vi "build_pck.vi"(8 "data in":u8[](array[numeric])=[0, 0, 0, 0], 9 "dev_id":u32, 10 "pck_num":u32, 11 "cmd_type":T1) -> (3 "w5500_pck":T2)   [LabVIEW 2021]
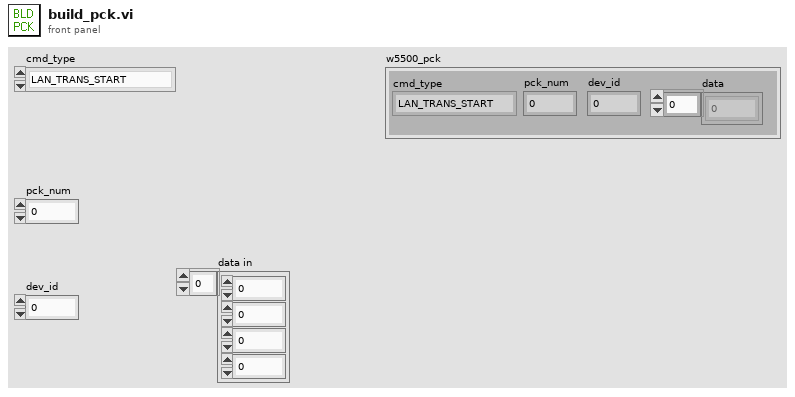
[diagram p1: front panel]
types:
  T1 = typedef "w5500_cmd.ctl" = enum32{"LAN_TRANS_START", "LAN_DATA_SZ", "LAN_CHUNK_SEND", "LAN_CHUNK_ACK", "LAN_DEVS_INFO", "LAN_DEVS_NUM", "LAN_DEVS_EXS", "LAN_DEVS_ACK", "LAN_CMD_ACK", "LAN_CMD_FIN", "LAN_SND_STAT", "LAN_REQ_STAT", "LAN_ANS_STAT", "LAN_ERR_STAT", "LAN_SETT_SET", "LAN_SETT_GET", "LAN_SETT_ACK", "LAN_SETT_ERR"}
  T2 = typedef "w5500_pck.ctl" = cluster{"cmd_type":T1, "pck_num":u32, "dev_id":u32, "data":u8[]}
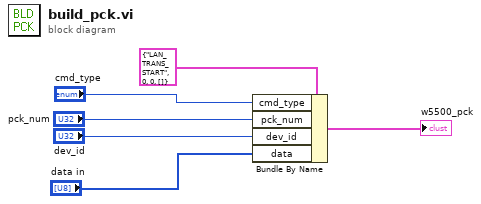
[diagram p0: block diagram]
diagram:
  n1 = Bundle By Name(cluster=T2 {"cmd_type"=enum."LAN_TRANS_START", "pck_num"=0, "dev_id"=0, "data"=[]} ("w5500_pck"), "cmd_type"="cmd_type", "pck_num"="pck_num", "dev_id"="dev_id", "data"="data in") -> (→"w5500_pck":T2)
